vi "Initial.vi"(7 "Serial Configuration":T1={"Baud Rate"=9600, "Parity"=0, "Stop Bits"=10, "Flow Control"=2} {"Flow Control" items=["None", "XON/XOFF", "RTS/CTS", "XON/XOFF & RTS/CTS", "DTR/DSR", "XON/XOFF & DTR/DSR"]; "Stop Bits" items=["1.0"=10, "1.5"=15, "2.0"=20]; "Parity" items=["None", "Odd", "Even", "Mark", "Space"]; "Baud Rate" items=["300"=300, "600"=600, "1200"=1200, "2400"=2400, "4800"=4800, "9600"=9600, "19200"=19200]}, 8 "error in (no error)":errorcluster, 9 "ID Query? (T: Yes)":bool=TRUE, 10 "Reset? (T: Yes)":bool=TRUE, 11 "EDUX1002G in":refnum<class "EDUX1002G.lvclass">) -> (0 "error out":errorcluster, 3 "EDUX1002G out":refnum<class "EDUX1002G.lvclass">)   [LabVIEW 2020, in "Osciloscope Tektronix.lvlib" / "EDUX1002G.lvclass"]
uses:
  EDUX1002G.lvclass
  C:/Users/Pablo/Osciloscope-Tek/TDS2000/Libraries/Osciloscope Tektronix/Clases/Osciloscope/Osciloscope.lvclass
  Clases/Osciloscope/Osciloscope.lvclass/Osciloscope.ctl
  Clases/Osciloscope/Read COM.vi
  <instrlib>/Agilent 2000 3000 X-Series/Agilent 2000 3000 X-Series.lvlib
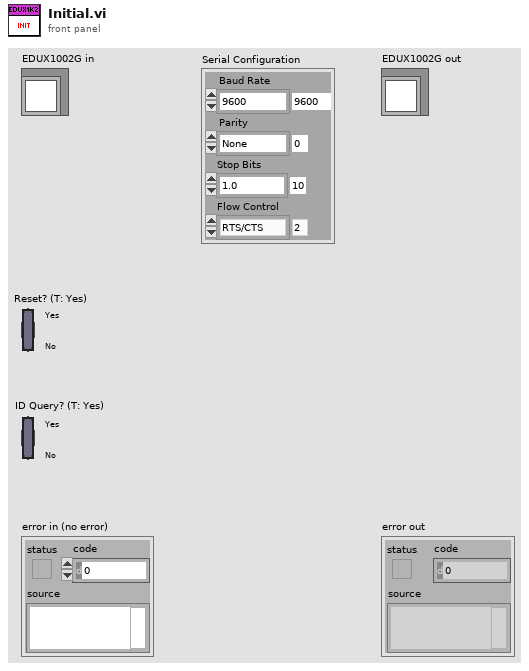
[diagram p1: front panel]
types:
  T1 = cluster{"Baud Rate":u32, "Parity":u16, "Stop Bits":u16, "Flow Control":u16}
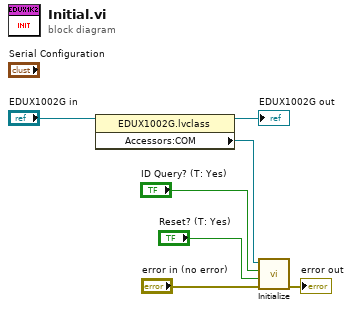
[diagram p0: block diagram]
diagram:
  n1 = property class="EDUX1002G.lvclass"(reference="EDUX1002G in") -> (reference out=→"EDUX1002G out":refnum<class "EDUX1002G.lvclass">, "Accessors:COM"=w1:refnum<visa-resource-name>)  [unwired: 1 in, 1 out]
  n2 = call <instrlib>:"Initialize.vi"("error in (no error)"="error in (no error)", "Reset (True)"="Reset? (T: Yes)", "ID Query (True)"="ID Query? (T: Yes)", "VISA resource name"=w1) -> ("error out"=→"error out":errorcluster)  [unwired: 6 in, 1 out]
